vi "ModuleDiedEvent.vi"() -> ()   [LabVIEW 2024]
uses:
  ModuleTemplates/NewTemplateModule/NewTemplate.lvclass
  RQMHCore/ModuleCore/Module.lvclass
  RQMHCore/ModuleCore/Show Front Panel.vi
  RQMHCore/Shared/Died.ctl
  RQMHCore/Shared/ModuleShared.lvlib
panel:
  out "Died":T1
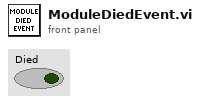
[diagram p1: front panel]
types:
  T1 = typedef "ModuleShared.lvlib/Died.ctl" = bool
  T2 = typedef "Module.lvclass/StandardBroadcasts.ctl" = cluster{"Died":refnum<user-event>, "Started":refnum<user-event>}
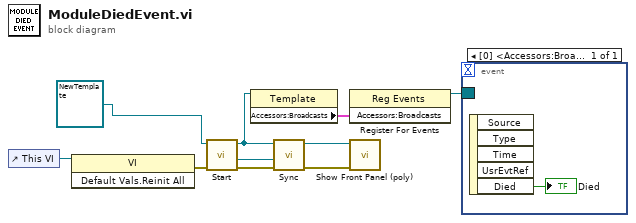
[diagram p0: block diagram]
diagram:
  n1 = control-ref of="This VI"() -> (w2:refnum<vi>)
  n2 = invoke class="VI" method="Default Vals.Reinit All"(reference=w2) -> (error out=w3:errorcluster)  [unwired: 2 in, 2 out]
  n3 = call "Start.vi"("error in (no error)"=w3, "JQMHCore in"=refnum<class "NewTemplate.lvclass"> refnum ("Template")) -> ("error out"=w6:errorcluster, "StartupHandshake out"=w7:refnum<class "ModuleStartup.lvclass">, "JQMHCore out"=w8:refnum<class "NewTemplate.lvclass">)  [unwired: 7 in]
  n4 = property class="Template"(reference=w8) -> ("Accessors:Broadcasts"=w10:T2)  [unwired: 1 in, 2 out]
  n5 = call "Sync.vi"("error in (no error)"=w6, "StartupHandshake out"=w7, "JQMHCore in"=w8) -> ("error out"=w4:errorcluster, "JQMHCore out"=w5:refnum<class "NewTemplate.lvclass">)  [unwired: 7 in]
  n6 = register-events(w10) -> (reference out=w9:refnum<event-registration>)  [unwired: 2 in, 1 out]
  n7 = call-poly "Show Front Panel (poly).vi"("error in (no error)"=w4, "JQMHCore in"=w5) -> ()  [unwired: 8 in, 2 out]
  n8 = event shown="[0] <Accessors:Broadcasts.Died>: User Event" {
    selector: w9 -> [_]
    dyn-events: _ -> [_]
    timeout: _ -> [_]
    event User Event {
      n9 = event-data() -> ("Died"=→"Died":T1)  [unwired: 1 in, 4 out]
    }
  }
